vi "Set Log Overwrite Method.vi"(8 "error in (no error)":errorcluster, 10 "Overwrite Method (0: Discard Newest)":i32(ring) items=["Discard Newest", "Discard Oldest"], 11 "VISA resource name":refnum<visa-resource-name>) -> (0 "error out":errorcluster, 3 "VISA resource name out":refnum<visa-resource-name>)   [LabVIEW 2015, in "Keithley 2600 Series.lvlib"]
doc: "Sets the event log overwrite method."
uses:
  Keithley 2600 Series.lvlib
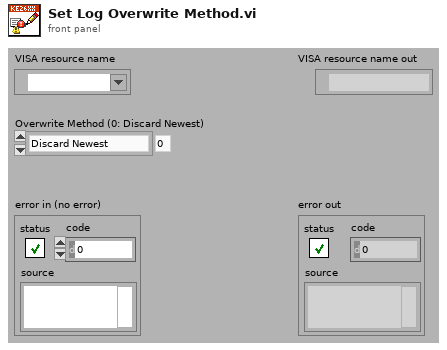
[diagram p1: front panel]
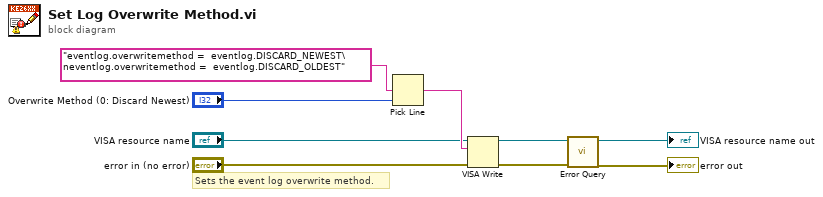
[diagram p0: block diagram]
diagram:
  # "Sets the event log overwrite method."
  n1 = Pick Line(multi-line string="eventlog.overwritemethod =  eventlog.DISCARD_NEWEST\neventlog.overwritemethod =  eventlog.DISCARD_OLDEST", line index="Overwrite Method (0: Discard Newest)") -> (output string=w7:string)  [unwired: 1 in]
  n2 = VISA Write(VISA resource name="VISA resource name", write buffer=w7, error in (no error)="error in (no error)") -> (VISA resource name out=w4:refnum<visa-resource-name>, error out=w3:errorcluster)  [unwired: 1 out]
  n3 = call "Error Query.vi"("error in (no error)"=w3, "VISA resource name"=w4) -> ("error out"=→"error out":errorcluster, "VISA resource name out"=→"VISA resource name out":refnum<visa-resource-name>)  [unwired: 6 in, 2 out]
